vi "List Mode - Seq - Configure Apparent Power Low Limitation.vi"(8 "error in (no error)":errorcluster, 10 "VA-LO":dbl min=0.0 max=4000.0, 11 "VISA resource name":refnum<visa-resource-name>) -> (0 "error out":errorcluster, 3 "VISA resource name out":refnum<visa-resource-name>)   [LabVIEW 2014, in "Associated Power Technologies 8500 Series.lvlib"]
doc: "Configure the apparent power (VA) low limitation in sequence.\n\nRange : 0 ~ max apparent power, 0 = OFF\n\n<B> Note : max apparent power</B>\nAPT-8505: 500VA\nAPT-8512: 1250VA\nAPT-8520: 2000VA\nAPT-8540: 4000VA\n\nDefault value: 0 (OFF)"
uses:
  <instrlib>/Associated Power Technologies 8500 Series/Associated Power Technologies 8500 Series.lvlib
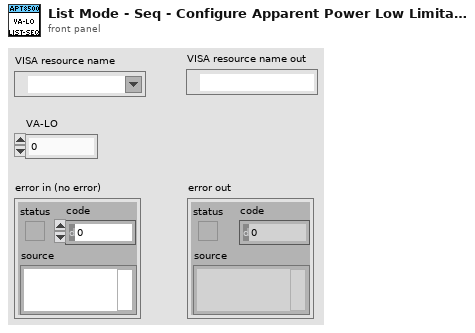
[diagram p1: front panel]
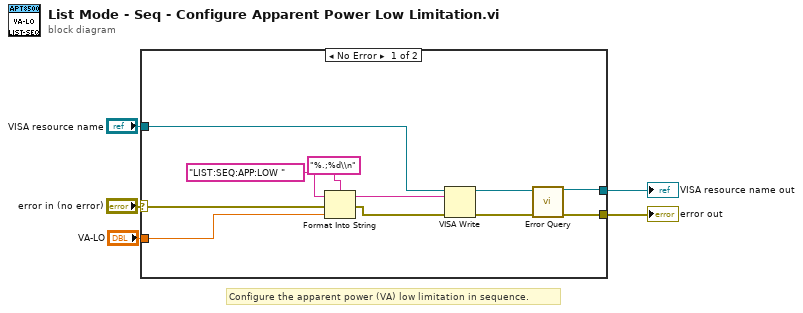
[diagram p0: block diagram]
diagram:
  # "Configure the apparent power (VA) low limitation in sequence."
  n1 = case shown="No Error" "error in (no error)" {
    selector: "error in (no error)" -> [w15 w17]
    tunnel: "VA-LO" -> [w16 _]
    tunnel: "VISA resource name" -> [w14 w18]
    tunnel: [w13 w18] -> w2
    tunnel: [w12 w17] -> w1
    frame No Error {
      n2 = Format Into String(format string="%.;%d\\n", initial string="LIST:SEQ:APP:LOW " ("command"), error in=w15, w16) -> (resulting string=w8:string, error out=w11:errorcluster)
      n3 = VISA Write(VISA resource name=w14, write buffer=w8, error in (no error)=w11) -> (VISA resource name out=w7:refnum<visa-resource-name>, error out=w6:errorcluster)  [unwired: 1 out]
      n4 = call <instrlib>:"Error Query.vi"("VISA resource name"=w7, "error in (no error)"=w6) -> ("VISA resource name out"=w13:refnum<visa-resource-name>, "error out"=w12:errorcluster)  [unwired: 10 in, 2 out]
    }
    frame Error {
    }
  }
  "VISA resource name out" <- w2
  "error out" <- w1
